vi "CCE MGLD PMJD PF SubVI010.vi"(1 "Q":dbl, 2 "u00":dbl, 3 "upq":dbl, 4 "P":dbl) -> (0 "npq":dbl)   [LabVIEW 2020]
doc: "Ceballos Conde Emanuel Meneses Gutiérrez Luis David Pineda Méndez Job Daniel 4MV6 Sistemas de visión artificial 2022/1 \nEste VI obtiene los momentos normalizados a partir de los parametros P,Q, upq, u00"
panel:
  # "Ceballos Conde Emanuel   -  Meneses Gutiérrez Luis David   -  Pineda Méndez Job Daniel 4MV6 Sistemas de visión artificial  2022/1             SubVI010"
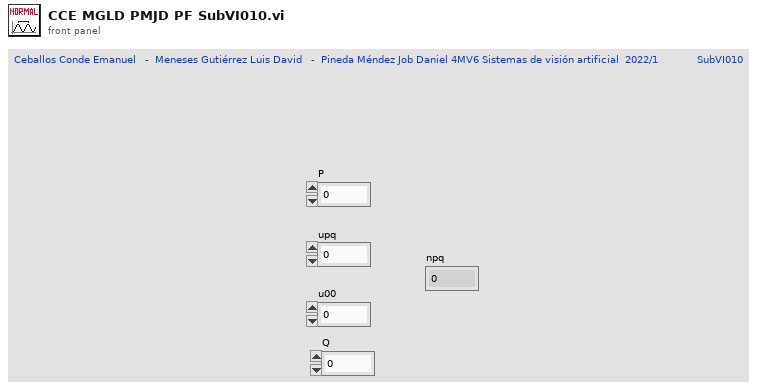
[diagram p1: front panel]
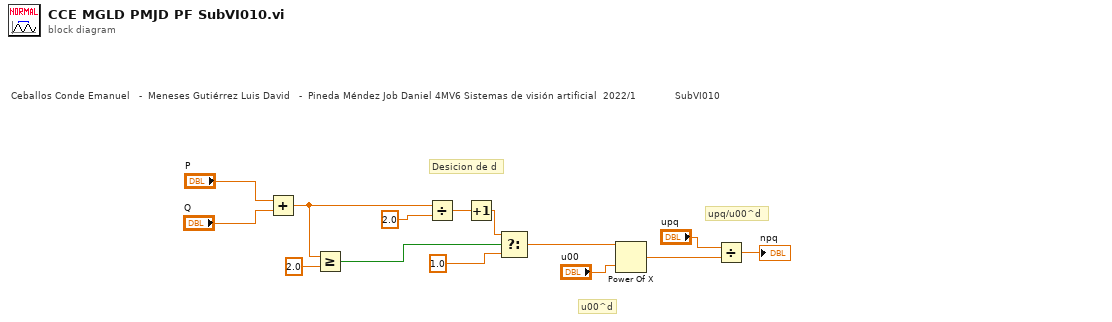
[diagram p0: block diagram]
diagram:
  # "Ceballos Conde Emanuel   -  Meneses Gutiérrez Luis David   -  Pineda Méndez Job Daniel 4MV6 Sistemas de visión artificial  2022/1             SubVI010"
  # "upq/u00^d"
  # "u00^d"
  # "Desicion de d"
  n1 = Add(x="P", y="Q") -> (x+y=w2:dbl)
  n2 = Greater Or Equal?(x=w2, y=2.0) -> (x >= y?=w3:bool)
  n3 = Divide(x=w2, y=2.0) -> (x/y=w6:dbl)
  n4 = Increment(x=w6) -> (x+1=w4:dbl)
  n5 = Select(t=w4, s=w3, f=1.0) -> (s? t:f=w1:dbl)
  n6 = Power Of X(1:"u00", 2:w1) -> (0:w9:dbl)
  n7 = Divide(x="upq", y=w9) -> (x/y=→"npq":dbl)
